vi "Compute LO Output Power Level.vi"(8 "error in":errorcluster, 11 "LO1 Frequency (Hz)":dbl format="%#_6p") -> (0 "error out":errorcluster, 3 "Power Level":dbl)   [LabVIEW 2017]
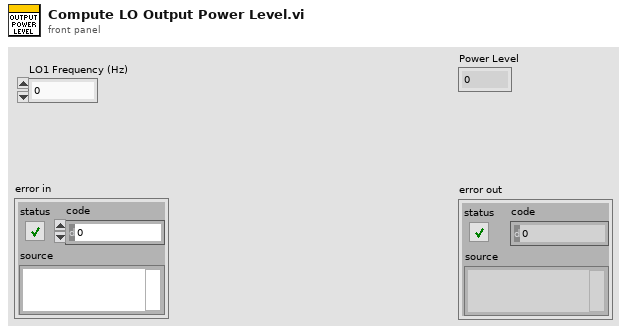
[diagram p1: front panel]
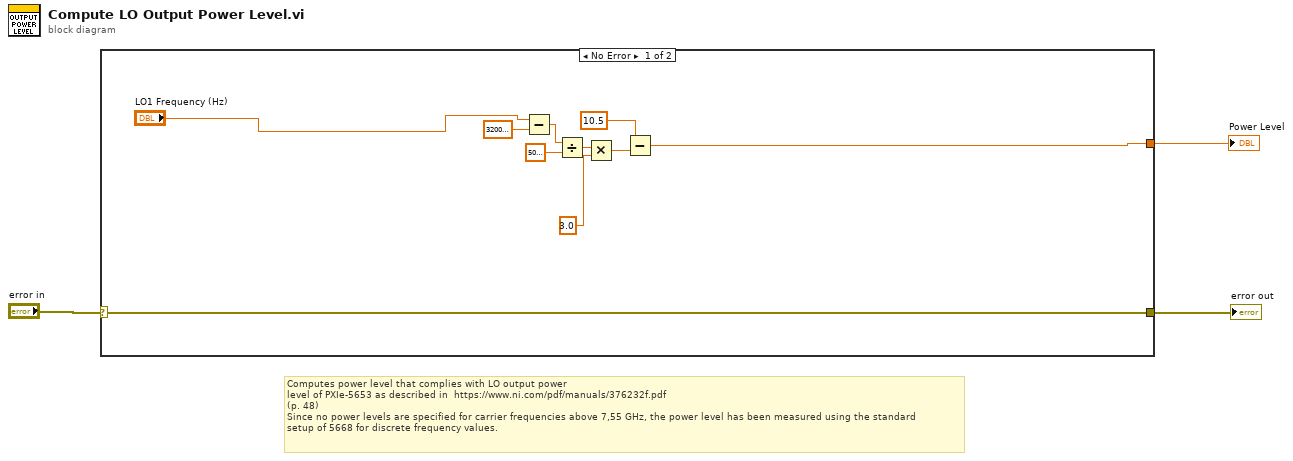
[diagram p0: block diagram]
diagram:
  # "Computes power level that complies with LO output power \nlevel of PXIe-5653 as described in  https://www.ni.com/pdf/manuals/376232f.pdf\n(p. 48)\nSince no power levels are specified for carrier frequencies above 7,55 GHz, the power level has been measured using the standard\nsetup of 5668 for discrete frequency values."
  n1 = case shown="No Error" "error in" {
    selector: "error in" -> [w11 w14]
    tunnel: [w13 _] -> w3
    tunnel: [w11 w14] -> w1
    frame No Error {
      n2 = Subtract(x="LO1 Frequency (Hz)", y=3200000000.0) -> (x-y=w5:dbl)
      n3 = Divide(x=w5, y=5000000000.0) -> (x/y=w7:dbl)
      n4 = Multiply(x=w7, y=3.0) -> (x*y=w9:dbl)
      n5 = Subtract(x=10.5, y=w9) -> (x-y=w13:dbl)
    }
    frame Error {
    }
  }
  "error out" <- w1
  "Power Level" <- w3
